vi "Configure Multipoint.vi"(8 "error in (no error)":errorcluster, 9 "Sample Count (1)":dbl=1.0 format="%#.6g", 10 "Trigger Type (0:Auto)":u16(ring) items=["Auto", "External", "Level", "Line", "Synchronous"], 11 "VISA resource name":refnum<visa-resource-name>) -> (0 "error out":errorcluster, 3 "VISA resource name out":refnum<visa-resource-name>)   [LabVIEW 2013, in "Agilent 3458.lvlib"]
doc: "Configures sample count, trigger type so as to enable multipoint functionality. \n\nNote: The user has the option of setting the trigger type only. The sample trigger type is set to \"AUTO\" and the trigger arm type is set to \"SGL\"(signal). That means that this instrument driver does not support \"HOLD\" and \"TIMER\" as trigger types."
uses:
  Agilent 3458.lvlib
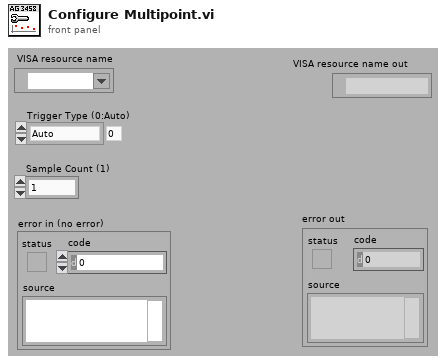
[diagram p1: front panel]
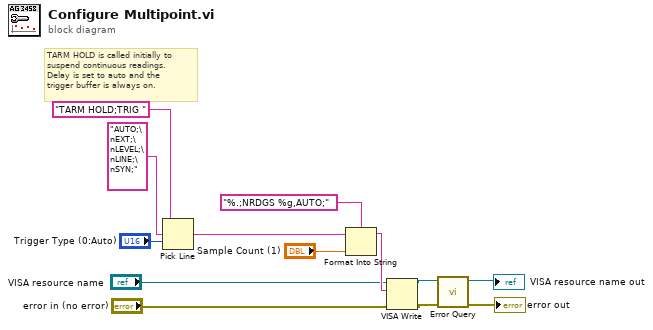
[diagram p0: block diagram]
diagram:
  # "TARM HOLD is called initially to \nsuspend continuous readings.\nDelay is set to auto and the \ntrigger buffer is always on."
  n1 = Pick Line(string ("")="TARM HOLD;TRIG ", multi-line string="AUTO;\nEXT;\nLEVEL;\nLINE;\nSYN;", line index="Trigger Type (0:Auto)") -> (output string=w9:string)
  n2 = Format Into String(format string="%.;NRDGS %g,AUTO;", initial string=w9, "Sample Count (1)") -> (resulting string=w8:string)  [unwired: 1 in, 1 out]
  n3 = VISA Write(VISA resource name="VISA resource name", write buffer=w8, error in (no error)="error in (no error)") -> (VISA resource name out=w4:refnum<visa-resource-name>, error out=w3:errorcluster)  [unwired: 1 out]
  n4 = call "Error Query.vi"("error in (no error)"=w3, "VISA resource name"=w4) -> ("error out"=→"error out":errorcluster, "VISA resource name out"=→"VISA resource name out":refnum<visa-resource-name>)  [unwired: 6 in, 2 out]
